vi "Test Correct Data is Sent When Setting DC Voltage.vi"(8 "error in (no error)":errorcluster, 11 "Test Case In":refnum<class "Low Level PSU Test.lvclass">) -> (0 "error out":errorcluster, 3 "Test Case Out":refnum<class "Low Level PSU Test.lvclass">)   [LabVIEW 2020, in "Low Level PSU With Tests.lvlib" / "Low Level PSU Test.lvclass"]
uses:
  Low Level PSU Test.lvclass
  C:/Program Files (x86)/National Instruments/LabVIEW 2020/vi.lib/Astemes/LUnit/Test Case.lvclass
  Mock Instrument Interface/Mock Instrument.lvclass
  C:/Git/astemes-gdevcon-2022/PSU Demo/Instrument Interface/Instrument Interface.lvclass
  Low Level PSU/Low Level PSU.lvclass
  <vilib>/Astemes/LUnit/Test Case.lvclass/Test Case.ctl
  01074fa8-ee8a-411d-bc8b-fc92c4f90959.vi
  <vilib>/Astemes/LUnit/Palette/Pass.vi
  <vilib>/Astemes/LUnit/Palette/Fail.vi
  <vilib>/Astemes/LUnit/Compare Variants.vi
  <vilib>/Astemes/LUnit/Describe Comparison.vi
  <vilib>/Astemes/LUnit/Set Assertion Type.vi
  <vilib>/Astemes/LUnit/Add test result.vi
  <vilib>/Astemes/LUnit/Variant to string.vi
  <vilib>/Astemes/LUnit/LUnit Record Assertion Result.vi
  <vilib>/Astemes/LUnit/LUnit Aggregate Assertion Results.vi
  <vilib>/Astemes/LUnit/Method Result/LUnit Merge Status.vi
  <vilib>/Astemes/LUnit/LUnit Concatenate result strings.vi
  <vilib>/Utility/Data Type/Get Type Information.vi
  <vilib>/Utility/LVClass/Get LV Class Name.vi
  Low Level PSU Test.lvclass/Low Level PSU Test.ctl
  C:/Git/astemes-gdevcon-2022/PSU Demo/Low Level PSU With Tests/Mock Instrument Interface/Mock Instrument.lvclass
  C:/Git/astemes-gdevcon-2022/PSU Demo/Low Level PSU With Tests/Instrument Interface/Instrument.lvclass
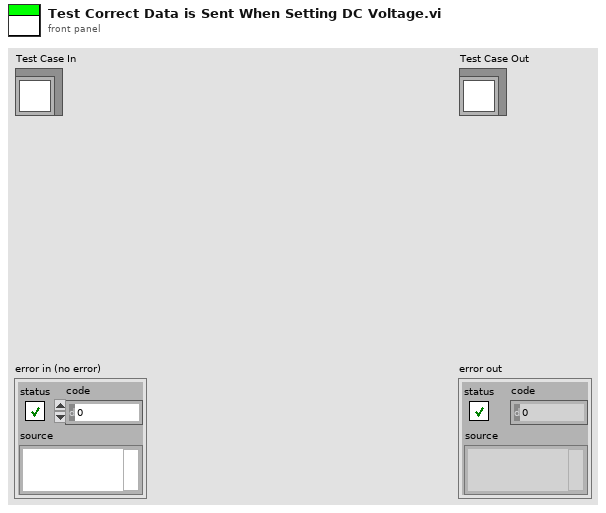
[diagram p1: front panel]
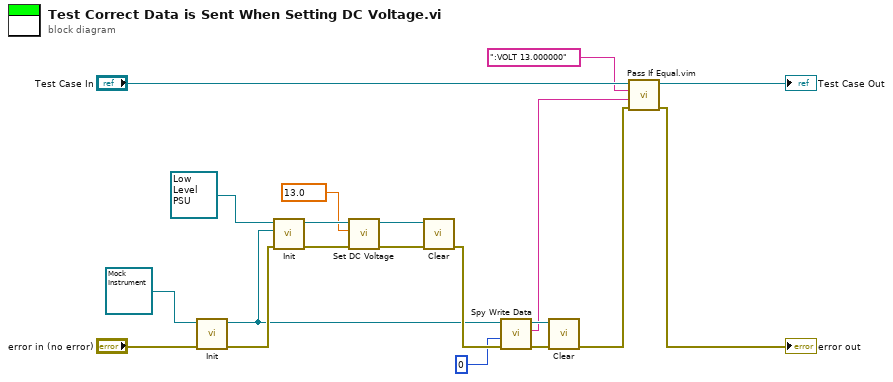
[diagram p0: block diagram]
diagram:
  n1 = call "Init.vi"("error in (no error)"="error in (no error)", "Mock Instrument Interface In"=refnum<class "Mock Instrument.lvclass"> refnum) -> ("error out"=w13:errorcluster, "Mock Instrument Interface Out"=w6:refnum<class "Mock Instrument.lvclass">)  [unwired: 8 in]
  n2 = call "Init.vi"("error in (no error)"=w13, "Instrument Interface"=w6, "Low Level PSU In"=refnum<class "Low Level PSU.lvclass"> refnum) -> ("error out"=w14:errorcluster, "Low Level PSU Out"=w15:refnum<class "Low Level PSU.lvclass">)  [unwired: 7 in]
  n3 = call "Set DC Voltage.vi"("error in (no error)"=w14, "Volt"=13.0, "Low Level PSU in"=w15) -> ("error out"=w10:errorcluster, "Low Level PSU out"=w11:refnum<class "Low Level PSU.lvclass">)  [unwired: 7 in]
  n4 = call "Clear.vi"("error in (no error)"=w10, "Low Level PSU In"=w11) -> ("error out"=w7:errorcluster)  [unwired: 8 in, 1 out]
  n5 = call "Spy Write Data.vi"("error in (no error)"=w7, "timeout in ms (-1)"=0, "Mock Instrument Interface in"=w6) -> ("error out"=w8:errorcluster, "Data"=w4:string, "Mock Instrument Interface out"=w9:refnum<class "Mock Instrument.lvclass">)  [unwired: 5 in, 1 out]
  n6 = call "Clear.vi"("error in (no error)"=w8, "Mock Instrument Interface In"=w9) -> ("error out"=w2:errorcluster)  [unwired: 8 in, 1 out]
  n7 = call "Pass If Equal.vim"("error in (no error)"=w2, "Actual"=w4, "Expected"=":VOLT 13.000000" ("Data"), "LUnit Test Case In"="Test Case In") -> ("error out"=→"error out":errorcluster, "LUnit Test Case Out"=→"Test Case Out":refnum<class "Low Level PSU Test.lvclass">)  [unwired: 6 in]
